vi "sim_scope.vi"(6 "amplitude":dbl=1.0 format="%#_13g", 7 "CHAN":T1={"channel name"="CHANNEL2", "probe attenuation"=1.0, "vertical offset"=0.0, "vertical range"=1.0, "vertical coupling"=1, "input impedance"=50.0} {"input impedance" format="%#_13g"; "vertical coupling" items=["AC", "DC", "GND"]; "vertical range" format="%.3f"; "vertical offset" format="%.3f"; "probe attenuation" format="%.3f"}, 8 "frequency":dbl=1000000.0 format="%#_13g", 9 "noise":dbl=0.1 format="%#_13g", 10 "dt":dbl=1e-08 format="%#_2e", 11 "Points":i32=1000) -> (2 "output waveform":waveform(dbl)={"t0"=timestamp(0 s since 1904-01-01), "dt"=1e-08, "Y"=array[1000 elements]})   [LabVIEW 2015, in "daq_simulate.lvlib"]
uses:
  daq_simulate.lvlib
  fake_oscilloscope/osc_channel.ctl
panel:
  out "min":dbl=-0.5
  out "max":dbl=0.5
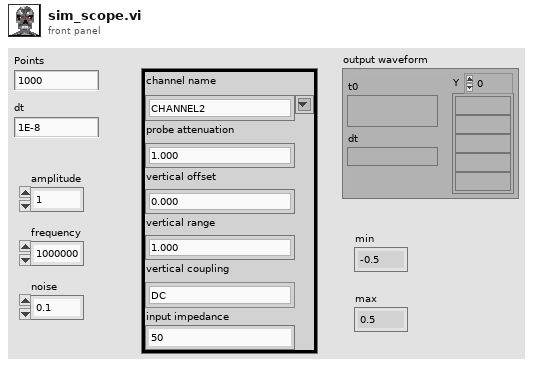
[diagram p1: front panel]
types:
  T1 = typedef "osc_channel.ctl" = cluster{"channel name":string, "probe attenuation":dbl, "vertical offset":dbl, "vertical range":dbl, "vertical coupling":i32, "input impedance":dbl}
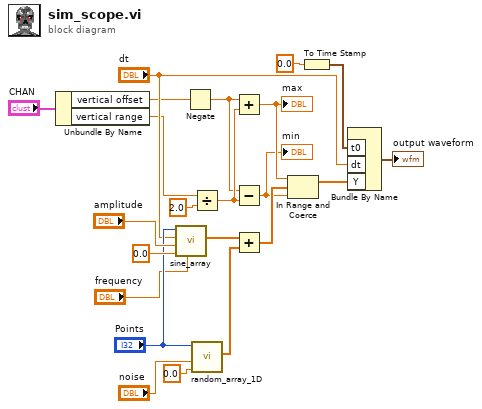
[diagram p0: block diagram]
diagram:
  n1 = Unbundle By Name("CHAN") -> ("vertical offset"=w6:dbl, "vertical range"=w9:dbl)
  n2 = call "sine_array.vi"("omega"="frequency", "offset"=0.0, "scale"="amplitude", "dx"="dt", "N"="Points") -> ("Array"=w20:dbl[])  [unwired: 6 in]
  n3 = Negate(x=w6) -> (-x=w5:dbl)
  n4 = Divide(x=w9, y=2.0) -> (x/y=w7:dbl)
  n5 = call "random_array_1D.vi"("offset"=0.0, "scale"="noise", "N"="Points") -> ("Array"=w21:dbl[])  [unwired: 8 in]
  n6 = Add(x=w5, y=w7) -> (x+y=w4:dbl)
  "max" <- w4
  n7 = Subtract(x=w5, y=w7) -> (x-y=w3:dbl)
  "min" <- w3
  n8 = Add(x=w20, y=w21) -> (x+y=w12:dbl[])
  n9 = In Range and Coerce(upper limit=w4, x=w12, lower limit=w3) -> (coerced(x)=w11:dbl[])  [unwired: 1 out]
  n10 = To Time Stamp(1:0.0 ("number")) -> (0:w22:timestamp)
  n11 = Bundle By Name("t0"=w22, "dt"="dt", "Y"=w11) -> (→"output waveform":waveform(dbl))  [unwired: 1 in]
